vi "Scan Setup.vi"(8 "error in (no error)":errorcluster, 11 "Magna Power Scan in":refnum<class "Magna Current Scan.lvclass">) -> (0 "error out":errorcluster, 3 "Magna Power Scan out":refnum<class "Magna Current Scan.lvclass">)   [LabVIEW 2017, in "Magna Current Scan.lvclass"]
doc: "Configure the Instrument based on the class member fields. This step comes after the user has closed the \"Scan Setup\" window and before the actual scan -- so instruments are configured with the user's specified settings."
uses:
  Magna Current Scan.lvclass
  Instruments/Magna-Power Power Supply/Magna Power.lvclass
  C:/LabVIEW-programs-dev/Instruments/Utility Classes/Scannable/Scannable.lvclass
  Scanner/Scanner.lvclass
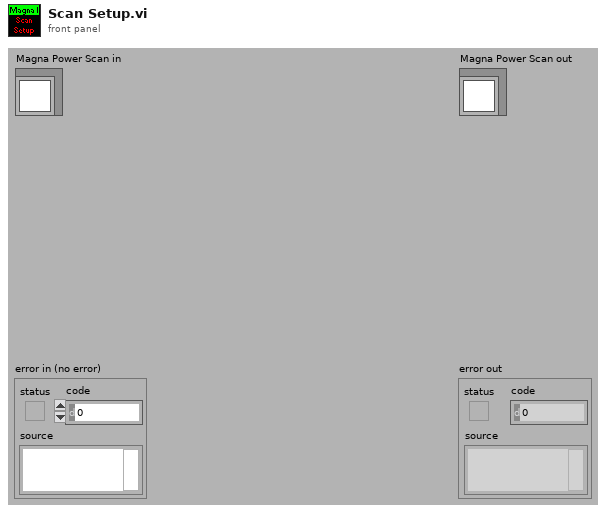
[diagram p1: front panel]
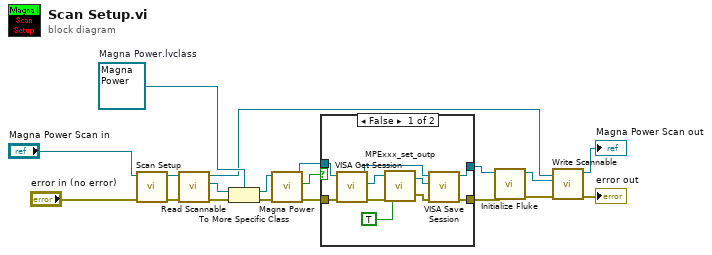
[diagram p0: block diagram]
diagram:
  w14 = refnum<class "Magna Power.lvclass"> refnum  # Magna Power.lvclass
  n1 = call-parent "Scan Setup.vi"("error in (no error)"="error in (no error)", "Scanner in"="Magna Power Scan in") -> ("error out"=w19:errorcluster, "Scanner out"=w18:refnum<class "Magna Current Scan.lvclass">)  [unwired: 8 in]
  n2 = call-dynamic "Read Scannable.vi"("error in (no error)"=w19, "Scanner.lvclass in"=w18) -> ("error out"=w17:errorcluster, "Scannable.lvclass"=w16:refnum<class "Scannable.lvclass">, "Scanner.lvclass out"=w3:refnum<class "Magna Current Scan.lvclass">)  [unwired: 7 in]
  n3 = To More Specific Class(target class=w14, reference=w16, error in=w17) -> (specific class reference=w13:refnum<class "Magna Power.lvclass">, error out=w15:errorcluster)
  n4 = call "Magna Power.vi"("error in (no error)"=w15, "Magna Power in"=w13) -> ("error out"=w7:errorcluster, "On?"=w8:bool, "Magna Power out"=w6:refnum<class "Magna Power.lvclass">)  [unwired: 7 in]
  n5 = case shown="False" w8 {
    tunnel: w7 -> [w29 w31]
    tunnel: [w27 w31] -> w4
    tunnel: w6 -> [w28 w30]
    tunnel: [w20 w30] -> w5
    frame False {
      n6 = call-dynamic "VISA Get Session.vi"("error in (no error)"=w29, "Instrument.lvclass in"=w28) -> ("error out"=w23:errorcluster, "VISA Resource Name"=w22:refnum<visa-resource-name>, "Instrument.lvclass out"=w21:refnum<class "Magna Power.lvclass">)  [unwired: 6 in, 1 out]
      n7 = call "MPExxx_set_outp.vi"("error in (no error)"=w23, "Output Control"=TRUE, "VISA session"=w22) -> ("error out"=w26:errorcluster, "dup VISA session"=w25:refnum<visa-resource-name>)
      n8 = call-dynamic "VISA Save Session.vi"("error in (no error)"=w26, "VISA Resource Name"=w25, "Instrument.lvclass in"=w21) -> ("error out"=w27:errorcluster, "Instrument.lvclass out"=w20:refnum<class "Magna Power.lvclass">)  [unwired: 7 in]
    }
    frame True {
    }
  }
  n9 = call "Initialize Fluke.vi"("error in (no error)"=w4, "Magna Power in"=w5) -> ("error out"=w2:errorcluster, "Magna Power out"=w1:refnum<class "Magna Power.lvclass">)  [unwired: 8 in]
  n10 = call-dynamic "Write Scannable.vi"("error in (no error)"=w2, "Scannable.lvclass"=w1, "Scanner.lvclass in"=w3) -> ("error out"=→"error out":errorcluster, "Scanner.lvclass out"=→"Magna Power Scan out":refnum<class "Magna Current Scan.lvclass">)  [unwired: 7 in]
